vi "test_TxGen-RxMon - Multiple Boards.vi"(8 "error in":errorcluster, 11 "reference in":refnum<class "AIM ARINC 664 Loopback.lvclass">) -> (0 "error out":errorcluster, 3 "reference out":refnum<class "AIM ARINC 664 Loopback.lvclass">)   [LabVIEW 2020, in "AIM ARINC 664 Loopback.lvclass"]
uses:
  AIM ARINC 664 Loopback.lvclass
  AIM ARINC 664 Loopback.lvclass/AIM ARINC 664 Loopback.ctl
  3f9c4eda-19e9-4962-b6bc-794414341bbb.vi
  6a3dd3ed-914d-4d14-bf18-724521aa5e28.vi
  56c9d474-e1ad-41d5-9732-7ebb07e8a0f2.vi
  <vilib>/NI VeriStand/Execution/Workspace/NI VeriStand - Get Multiple Channel Values.vi
  NationalInstruments.VeriStand.SystemDefinitionAPI
  <vilib>/addons/_JKI Toolkits/VI Tester/TestCase.llb/TestCase.lvclass
  <vilib>/NI VeriStand/Execution/Workspace/NI_VS Workspace ExecutionAPI.lvlib
  Scripting/AIM ARINC 664 Scripting.lvlib
  Import/AIM ARINC 664 Import.lvlib
  C:/Program Files/National Instruments/LabVIEW 2024/vi.lib/addons/_JKI Toolkits/VI Tester/TestCase.llb/TestCase.lvclass
panel:
  out "Elapsed Time (s)":dbl
  out "Values":dbl[](array[numeric])
  in  "tolerance (5 samples)":dbl=20.0 caption="Time Target (s)"
  in  "Time Target (s)":dbl=5.0
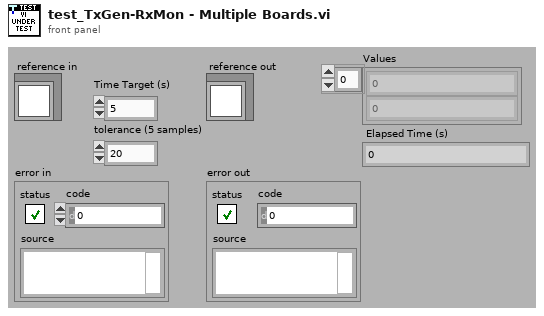
[diagram p1: front panel]
types:
  T1 = typedef "Custom Device API.lvlib/Custom Device Item Ref.ctl" = u64
  T2 = typedef "AIM ARINC 664 Import.lvlib/Board Top Level Configuration.ctl" = cluster{"boardSetup":T3, "portConfiguration":T4[]}
  T3 = typedef "AIM ARINC 664 Import.lvlib/board_setup.ctl" = cluster{"boardId":u32, "portSpeed":u32, "portConfig":u32}
  T4 = typedef "AIM ARINC 664 Import.lvlib/port_configuration.ctl" = cluster{"portSetup":T5, "Tx_Generic":T6[], "Rx_Monitor":cluster{"DefaultCronoMode":u32, "GlbMonBufferSizeIn":u32, "CaptureMode":u32, "MaxFileSizeMB":u32, "Strobe":u32, "TriggerPosition":u32}[], "Tx_UDP":cluster{"tx_udp_setup":cluster{"VlId":i32, "Bag":i32, "NetSelect":u32, "domainID":u8, "sideID":u8, "locationID":u8, "interfaceID":u8, "NumOfSubVl":u16, "Skew":u32, "MaxFrameLength":u32, "FrameBufferSize":u32}, "commPorts":T14[], "sapPorts":T15[]}[], "Rx_UDP":cluster{"Tx_UDP":T16, "commPorts":T17[], "sapPorts":T18[]}[]}
  T5 = typedef "AIM ARINC 664 Import.lvlib/port_setup.ctl" = cluster{"port Id":u32, "redundant":bool}
  T6 = typedef "AIM ARINC 664 Import.lvlib/session_tx_generic.ctl" = cluster{"tx_generic_setup":T7, "Frame Headers":T8[]}
  T7 = typedef "AIM ARINC 664 Import.lvlib/tx_generic_setup.ctl" = cluster{"QueueSizeIn":u32, "Count":i32, "StartMode":i32}
  T8 = typedef "AIM ARINC 664 Import.lvlib/frame_tx_generic.ctl" = cluster{"FrameID":string, "PayloadID":string, "Frame header":cluster{"FrameStartMode":i32, "InterFrameGap":i32, "PacketGroupWaitTime":i32, "NetSelect":u32, "PayloadBufferMode":i32, "PayloadGenerationMode":i32, "PhysErrorInjection":i32, "PreambleCount":i32, "SequenceNumberInit":T9, "SequenceNumberOffset":T10, "Skew":i32}, "Parameters":T11[]}
  T9 = typedef "AIM ARINC 664 Import.lvlib/frame_tx_generic_seqNumberInit.ctl" = i32
  T10 = typedef "AIM ARINC 664 Import.lvlib/frame_tx_generic_seqNumberOffset.ctl" = i32
  T11 = typedef "AIM ARINC 664 Import.lvlib/frame_parameter.ctl" = cluster{"name":string, "default value":dbl, "unit":string, "Parameter":T12}
  T12 = typedef "AIM ARINC 664 Import.lvlib/frame_parameter_definition.ctl" = cluster{"start index":i32, "size":i32, "encoding":T13, "signed":bool, "scale multiplier":dbl, "scale offset":dbl}
  T13 = typedef "Encoding (Arinc664).ctl" = u16
  T14 = typedef "AIM ARINC 664 Import.lvlib/port_tx_udp_comm.ctl" = cluster{"PayloadID":string, "partitionID":u8, "UdpSrcPort":u16, "UdpDstPort":u16, "PortType":enum16{"FDX_UDP_SAMPLING", "FDX_UDP_QUEUING"}, "SubVIId":u32, "UdpNumBufMessages":u32, "UdpMaxMessageSize":u32, "UdpSamplingRate":u32, "Parameters":T11[]}
  T15 = typedef "AIM ARINC 664 Import.lvlib/port_tx_udp_sap.ctl" = cluster{"PayloadID":string, "SubVlId":u8, "UdpSrcPort":u16, "UdpNumBufMessages":u32, "UdpMaxMessageSize":u32, "partitionID":u8, "domainID":u8, "sideID":u8, "locationID":u8, "interfaceID":u8, "Parameters":T11[]}
  T16 = typedef "AIM ARINC 664 Import.lvlib/rx_udp_setup.ctl" = cluster{"VerificationMode":u32, "Bag":u32, "Jitter":u32, "MaxFrameLength":u32, "MaxSkew":u32, "VLBufSize":u32, "FilterMode":u32, "FilterPosition":u32, "Padding":u32, "FilterMask":u32, "FilterData":u32, "MinFrameLength":u32, "VlId":u16, "VLRange":u32}
  T17 = typedef "AIM ARINC 664 Import.lvlib/port_rx_udp_comm.ctl" = cluster{"PayloadID":string, "domainID":u8, "sideID":u8, "locationID":u8, "partitionID":u8, "UdpSrcPort":u16, "UdpDstPort":u16, "PortType":enum16{"FDX_UDP_SAMPLING", "FDX_UDP_QUEUING"}, "SubVIId":u32, "UdpNumBufMessages":u32, "UdpMaxMessageSize":u32, "UdpSamplingRate":u32, "Parameters":T11[]}
  T18 = typedef "AIM ARINC 664 Import.lvlib/port_rx_udp_sap.ctl" = cluster{"PayloadID":string, "UdpDstPort":u16, "UdpNumBufMessages":u32, "UdpMaxMessageSize":u32, "Parameters":T11[]}
  T19 = typedef "Payload Map.ctl" = map{string, T20}
  T20 = typedef "Payload Record Type.ctl" = cluster{"Data":u8[], "Type of Frame":T21}
  T21 = typedef "Type of Payload.ctl" = u16
  T22 = typedef "NI_VS Workspace ExecutionAPI.lvlib/WorkspaceAPI.ctl" = refnum<k24>
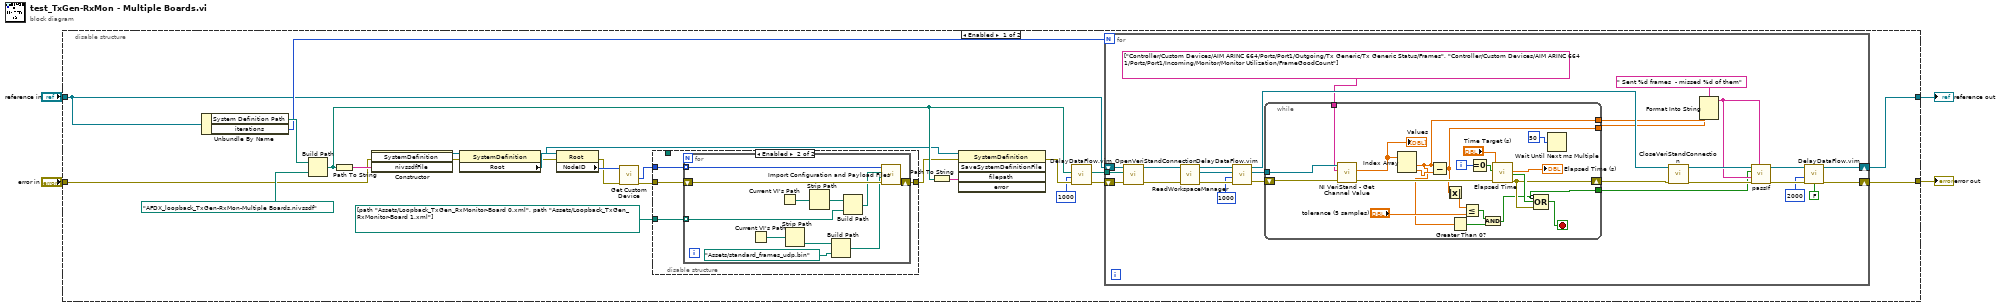
[diagram p0: block diagram]
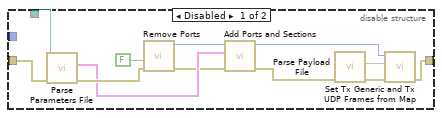
[diagram p2: hidden frame]
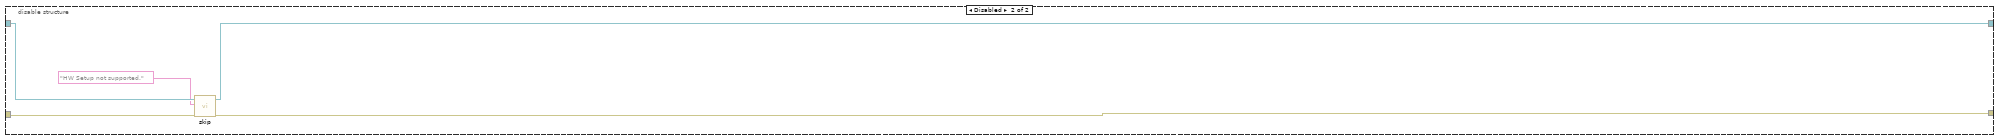
[diagram p3: hidden frame]
diagram:
  n1 = disable-structure shown="Enabled" {
    disable-tunnel: "reference in" -> [w7 w107]
    disable-tunnel: "error in" -> [w8 w106]
    disable-tunnel: [w28 w105] -> w2
    disable-tunnel: [w27 w104] -> w1
    frame Enabled {
      n2 = Unbundle By Name(w7) -> ("System Definition Path"=w26:path, "iterations"=w12:i32)
      n3 = Build Path(base path=w26, name or relative path=path "AFDX_loopback_TxGen-RxMon-Multiple Boards.nivssdf") -> (appended path=w23:path)
      n4 = Path To String(path=w23) -> (string=w24:string)
      n5 = constructor class="SystemDefinition"(error in=w8, "nivssdfFile"=w24) -> (reference out=w22:refnum<k24>, error out=w20:errorcluster)  [unwired: 2 in, 2 out]
      n6 = property class="SystemDefinition"(reference=w22, error in=w20) -> (reference out=w17:refnum<k24>, error out=w19:errorcluster, "Root"=w21:refnum<k24>)
      n7 = property class="Root"(reference=w21, error in=w19) -> (error out=w14:errorcluster, "NodeID"=w15:u64)  [unwired: 1 out]
      n8 = call "Get Custom Device.vi"("error in"=w14, "custom device ref in"=w15) -> ("error out"=w13:errorcluster, "Item Refs"=w5:T1[])  [unwired: 5 in, 3 out]
      n9 = disable-structure shown="Enabled" {
        disable-tunnel: w13 -> [w78 w91]
        disable-tunnel: _ -> [w75 _]
        disable-tunnel: [w74 w90] -> w18
        disable-tunnel: path[] [path "Assets/Loopback_TxGen_RxMonitor-Board 0.xml", path "Assets/Loopback_TxGen_RxMonitor-Board 1.xml"] -> [_ w89]
        disable-tunnel: w5 -> [_ w88]
        frame Disabled {
          n10 = call "Parse Parameters File.vi"("error in"=w78, "path to XML document"=w75) -> ("error out"=w87:errorcluster, "board configuration out"=w84:T2)  [unwired: 7 in, 1 out]
          n11 = call "Remove Ports.vi"("error in"=w87, "refresh?"=FALSE) -> ("error out"=w83:errorcluster, "Custom device Ref out"=w85:T1, "Custom device Ref"=w86:T1)  [unwired: 7 in]
          n12 = call "Add Ports and Sections.vi"("error in"=w83, "board configuration in"=w84, "custom device ref"=w85) -> ("error out"=w82:errorcluster, "custom device ref out"=w77:T1)  [unwired: 7 in]
          n13 = call "Parse Payload File.vi"("error in"=w82) -> ("error out"=w81:errorcluster, "Map"=w80:T19, "frame array path in"=w76:path)  [unwired: 7 in, 1 out]
          n14 = call "Set Tx Generic and Tx UDP Frames from Map.vi"("error in"=w81, "payload map"=w80, "custom device ref"=w77) -> ("error out"=w74:errorcluster)  [unwired: 7 in, 1 out]
        }
        frame Enabled {
          n15 = for {
            shift-right: [w101] -> w90
            shift-left: w91 -> [w102]
            tunnel: w89 -> [w93] mode=indexing
            tunnel: w88 -> [w92] mode=indexing
            n16 = Current VI's Path() -> (path=w98:path)
            n17 = Current VI's Path() -> (path=w95:path)
            n18 = Strip Path(path=w98) -> (stripped path=w100:path)  [unwired: 1 out]
            n19 = Strip Path(path=w95) -> (stripped path=w96:path)  [unwired: 1 out]
            n20 = Build Path(base path=w100, name or relative path=path "Assets/standard_frames_udp.bin") -> (appended path=w97:path)
            n21 = Build Path(base path=w96, name or relative path=w93) -> (appended path=w94:path)
            n22 = call "Import Configuration and Payload Files.vi"("error in"=w102, "payload file path"=w97, "parameters configuration file path"=w94, "custom device ref"=w92) -> ("error out"=w101:errorcluster)  [unwired: 6 in, 1 out]
          }
        }
      }
      n23 = Path To String(path=w23) -> (string=w16:string)
      n24 = invoke class="SystemDefinition" method="SaveSystemDefinitionFile"(reference=w17, error in=w18, "filepath"=w16) -> (error out=w11:errorcluster)  [unwired: 2 in, 4 out]
      n25 = call "DelayDataFlow.vim"("value in"=w11, "milliseconds to wait"=u32 1000) -> ("value out"=w10:errorcluster)  [unwired: 2 in, 1 out]
      n26 = for {
        N: w12 -> [_]
        tunnel: w23 -> [w34]
        shift-right: [w51] -> w27
        shift-left: w7 -> [w52]
        shift-right: [w32] -> w28
        shift-left: w10 -> [w35]
        n27 = call-dynamic "OpenVeriStandConnection.vi"("error in (no error)"=w35, "System Definition File"=w34, "VeriStand Test Case in"=w52) -> ("error out"=w50:errorcluster, "VeriStand Test Case out"=w45:refnum<class "AIM ARINC 664 Loopback.lvclass">)  [unwired: 6 in, 1 out]
        n28 = call-dynamic "ReadWorkspaceManager.vi"("error in (no error)"=w50, "VeriStand Test Case in"=w45) -> ("error out"=w40:errorcluster, "Workspace"=w43:T22, "VeriStand Test Case out"=w44:refnum<class "AIM ARINC 664 Loopback.lvclass">)  [unwired: 7 in]
        n29 = call "DelayDataFlow.vim"("value in"=w40, "milliseconds to wait"=u32 1000) -> ("value out"=w39:errorcluster)  [unwired: 2 in, 1 out]
        n30 = while {
          tunnel: w43 -> [w73]
          shift-right: [w66] -> w42
          shift-left: w39 -> [w71]
          tunnel: [w59] -> w41
          tunnel: [w58] -> w37
          tunnel: [w57] -> w36
          tunnel: string[] ["Controller/Custom Devices/AIM ARINC 664/Ports/Port1/Outgoing/Tx Generic/Tx Generic Status/Frames", "Controller/Custom Devices/AIM ARINC 664 1/Ports/Port1/Incoming/Monitor/Monitor Utilization/FrameGoodCount"] ("Channels") -> [w55]
          i -> [w54]
          stop <- w68 stop-if-true
          n31 = call-poly <vilib>:"NI VeriStand - Get Channel Value.vi"("error in (no error)"=w71, "Channels"=w55, "WorkspaceManager in"=w73) -> ("error out"=w70:errorcluster, "Values"=w65:dbl[])  [unwired: 6 in, 1 out]
          "Values" <- w65
          n32 = Index Array(array=w65) -> (element #1=w58:dbl, element #2=w64:dbl)  [unwired: 2 in]
          n33 = Subtract(x=w58, y=w64) -> (x-y=w57:dbl)
          n34 = Absolute Value(x=w57) -> (abs(x)=w63:dbl)
          n35 = Greater Than 0?(x=w58) -> (x > 0?=w60:bool)
          n36 = Less Or Equal?(x=w63, y="tolerance (5 samples)") -> (x <= y?=w61:bool)
          n37 = Equal To 0?(x=w54) -> (x = 0?=w53:bool)
          n38 = And(x=w61, y=w60) -> (x .and. y?=w59:bool)
          n39 = call "Elapsed Time"("Time Target (s)"="Time Target (s)", "Reset"=w53, "error in (no error)"=w70) -> ("Elapsed Time (s)"=→"Elapsed Time (s)":dbl, "Time has Elapsed"=w69:bool, "error out"=w66:errorcluster)  [unwired: 9 in, 5 out]
          n40 = Compound Arithmetic op=OR(invert w59, w69, w66) -> (w68:bool)
          n41 = Wait Until Next ms Multiple(millisecond multiple=u32 50 ("millisecond timer value")) -> ()  [unwired: 1 out]
        }
        n42 = call-dynamic "CloseVeriStandConnection.vi"("error in (no error)"=w42, "VeriStand Test Case in"=w44) -> ("error out"=w49:errorcluster, "VeriStand Test Case out"=w48:refnum<class "AIM ARINC 664 Loopback.lvclass">)  [unwired: 8 in]
        n43 = Format Into String(format string=" Sent %d frames  - missed %d of them", w37, w36) -> (resulting string=w46:string)  [unwired: 2 in, 1 out]
        n44 = call-dynamic "passIf.vi"("custom report message (\"\")"=w46, "error in (no error)"=w49, "message (\"\")"=w46, "pass"=w41, "TestCase in"=w48) -> ("error out"=w31:errorcluster, "TestCase out"=w51:refnum<class "AIM ARINC 664 Loopback.lvclass">)  [unwired: 5 in]
        n45 = call "DelayDataFlow.vim"("value in"=w31, "milliseconds to wait"=u32 2000, "no delay on error (T)"=FALSE) -> ("value out"=w32:errorcluster)  [unwired: 1 in, 1 out]
      }
    }
    frame Disabled {
      n46 = call <vilib>:"skip.vi"("error in (no error)"=w106, "skipMessage"="HW Setup not supported.", "TestCase in"=w107) -> ("error out"=w105:errorcluster, "TestCase out"=w104:refnum<class "AIM ARINC 664 Loopback.lvclass">)  [unwired: 7 in]
    }
  }
  "error out" <- w2
  "reference out" <- w1
